vi "Get Name.vi"(8 "error in (no error)":errorcluster, 11 "EL-Go To Height in":refnum<class "EL-Go To Height.lvclass">) -> (0 "error out":errorcluster, 2 "Command Name":string, 3 "EL-Go To Height out":refnum<class "EL-Go To Height.lvclass">)   [LabVIEW 2014, in "Elevator.lvlib" / "EL-Go To Height.lvlib" / "EL-Go To Height.lvclass"]
uses:
  EL-Go To Height.lvclass
  Robot Actor Framework/Command Actor/Command Actor Class/Command Actor.lvclass
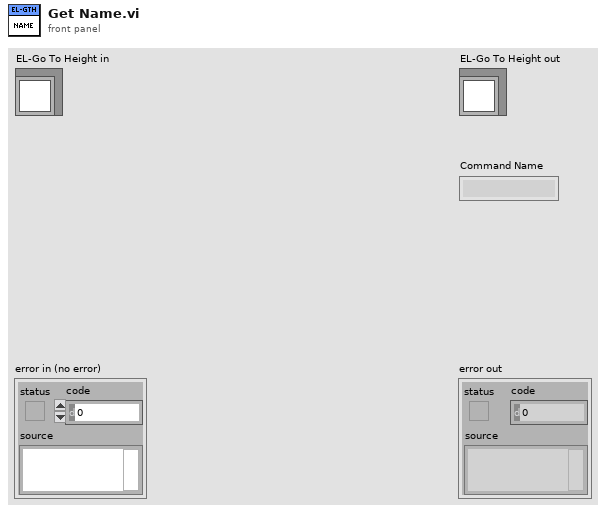
[diagram p1: front panel]
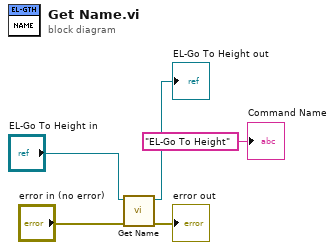
[diagram p0: block diagram]
diagram:
  n1 = call-parent "Get Name.vi"("error in (no error)"="error in (no error)", "Command Actor in"="EL-Go To Height in") -> ("error out"=→"error out":errorcluster, "Command Actor out"=→"EL-Go To Height out":refnum<class "EL-Go To Height.lvclass">)  [unwired: 7 in, 1 out]
  "Command Name" <- "EL-Go To Height" ("Command Name")
